vi "SCE_create_border.vi"(7 "VIC-II":T1, 11 "screen in":picture) -> (3 "screen out":picture)   [LabVIEW 2018]
uses:
  SCE_VIC-II_registry.ctl
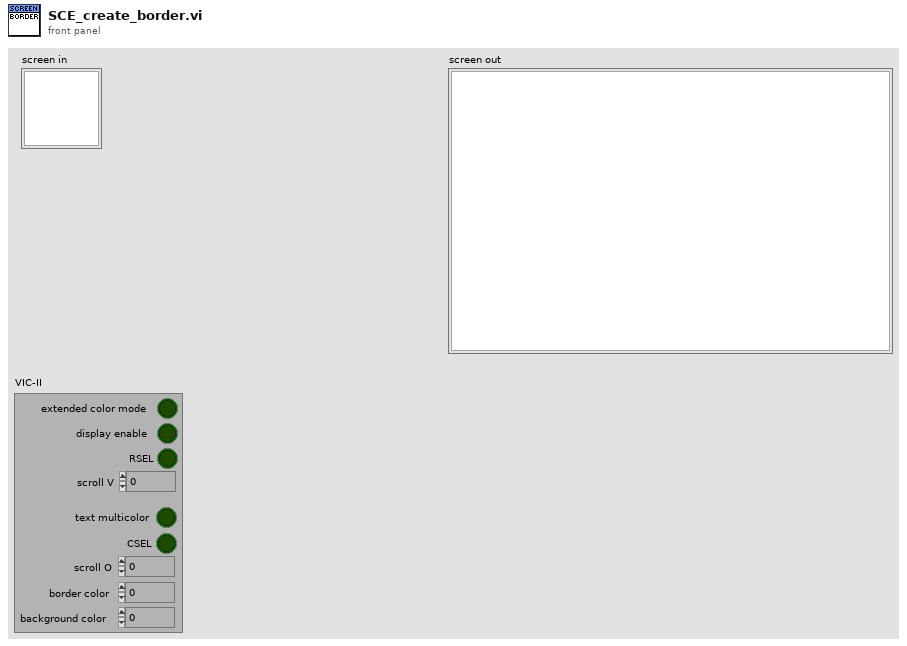
[diagram p1: front panel]
types:
  T1 = typedef "SCE_VIC-II_registry.ctl" = cluster{"extended color mode":bool, "display enable":bool, "RSEL":bool, "scroll V":u8, "text multicolor":bool, "CSEL":bool, "scroll O":u8, "border color":u8, "background color":u8}
  T2 = cluster{"left":i16, "top":i16, "right":i16, "bottom":i16}
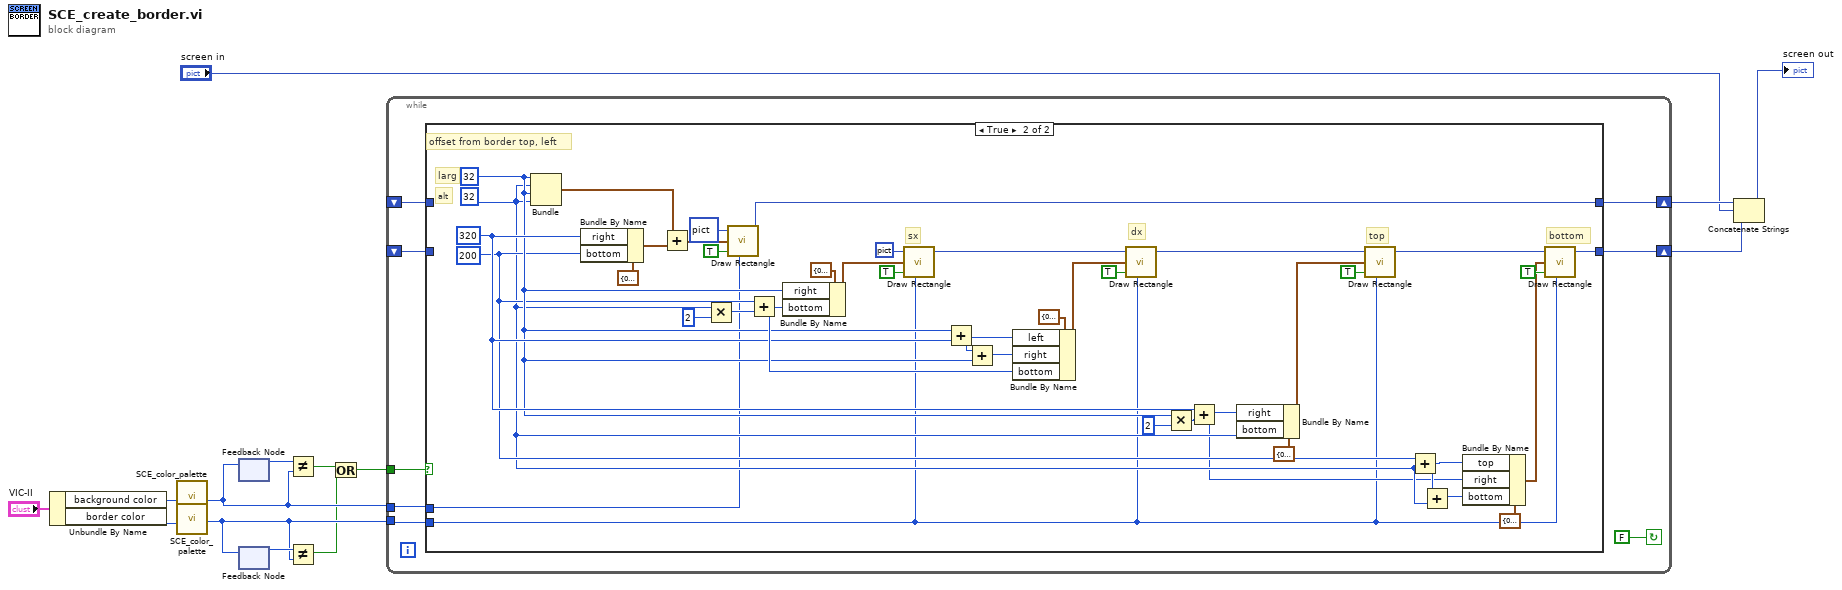
[diagram p0: block diagram]
diagram:
  n1 = Unbundle By Name("VIC-II") -> ("background color"=w13:u8, "border color"=w12:u8)
  n2 = call "SCE_color_palette.vi"("color index"=w13) -> ("selected color"=w6:u32)  [unwired: 9 in, 1 out]
  n3 = call "SCE_color_palette.vi"("color index"=w12) -> ("selected color"=w4:u32)  [unwired: 9 in, 1 out]
  n4 = feedback-in #1(w6) -> ()
  n5 = feedback #1() -> (w7:u32)  [unwired: 1 in]
  n6 = feedback #2() -> (w5:u32)  [unwired: 1 in]
  n7 = feedback-in #2(w4) -> ()
  n8 = Not Equal?(x=w7, y=w6) -> (x != y?=w3:bool)
  n9 = Not Equal?(x=w5, y=w4) -> (x != y?=w2:bool)
  n10 = Or(x=w3, y=w2) -> (x .or. y?=w1:bool)
  n11 = while {
    tunnel: w6 -> [w20]
    tunnel: w4 -> [w19]
    shift-right: [w22] -> w11
    shift-left: _ -> [w16]
    shift-right: [w21] -> w8
    shift-left: _ -> [w15]
    tunnel: w1 -> [w17]
    stop <- FALSE continue-if-true
    n12 = case shown="True" w17 {
      tunnel: [w24 w61] -> w22
      tunnel: [w23 w27] -> w21
      tunnel: w20 -> [_ w26]
      tunnel: w19 -> [_ w25]
      tunnel: w16 -> [w24 _]
      tunnel: w15 -> [w23 _]
      frame False {
      }
      frame True {
        w43 = i16 320 ("right")
        w32 = i16 200 ("bottom")
        w30 = i16 32 ("x")
        w40 = i16 32 ("x")
        # "bottom"
        # "top"
        # "dx"
        # "sx"
        # "alt"
        # "larg"
        # "offset from border top, left"
        n13 = Bundle("x"=w40, "x"=w30, "x"=w40, "x"=w30) -> (w64:cluster{"x":i16, "x":i16, "x":i16, "x":i16})  [unwired: 1 in]
        n14 = Bundle By Name(cluster=T2 {"left"=0, "top"=0, "right"=320, "bottom"=200} ("rect"), "right"=w43, "bottom"=w32) -> (w58:T2)
        n15 = Add(x=w64, y=w58) -> (x+y=w63:cluster{i16, i16, i16, i16})
        n16 = Multiply(x=w30, y=i16 2) -> (x*y=w47:i16)
        n17 = call <vilib>:"Draw Rectangle.vi"("picture"=picture data[5B], "rect"=w63, "fill?(F)"=TRUE, "color(black)"=w26) -> ("new picture"=w61:picture)  [unwired: 5 in]
        n18 = Add(x=w32, y=w47) -> (x+y=w45:i16)
        n19 = Bundle By Name(cluster=T2 {"left"=0, "top"=0, "right"=320, "bottom"=200} ("rect"), "right"=w40, "bottom"=w45) -> (w56:T2)
        n20 = call <vilib>:"Draw Rectangle.vi"("picture"=picture data[5B], "rect"=w56, "fill?(F)"=TRUE, "color(black)"=w25) -> ("new picture"=w50:picture)  [unwired: 5 in]
        n21 = Add(x=w40, y=w43) -> (x+y=w49:i16)
        n22 = Add(x=w49, y=w40) -> (x+y=w48:i16)
        n23 = Bundle By Name(cluster=T2 {"left"=0, "top"=0, "right"=320, "bottom"=200} ("rect"), "left"=w49, "right"=w48, "bottom"=w45) -> (w52:T2)
        n24 = call <vilib>:"Draw Rectangle.vi"("picture"=w50, "rect"=w52, "fill?(F)"=TRUE, "color(black)"=w25) -> ("new picture"=w37:picture)  [unwired: 5 in]
        n25 = Multiply(x=w40, y=i16 2) -> (x*y=w41:i16)
        n26 = Add(x=w43, y=w41) -> (x+y=w28:i16)
        n27 = Bundle By Name(cluster=T2 {"left"=0, "top"=0, "right"=320, "bottom"=200} ("rect"), "right"=w28, "bottom"=w30) -> (w39:T2)
        n28 = call <vilib>:"Draw Rectangle.vi"("picture"=w37, "rect"=w39, "fill?(F)"=TRUE, "color(black)"=w25) -> ("new picture"=w35:picture)  [unwired: 5 in]
        n29 = Add(x=w32, y=w30) -> (x+y=w31:i16)
        n30 = Add(x=w31, y=w30) -> (x+y=w29:i16)
        n31 = Bundle By Name(cluster=T2 {"left"=0, "top"=0, "right"=320, "bottom"=200} ("rect"), "top"=w31, "right"=w28, "bottom"=w29) -> (w33:T2)
        n32 = call <vilib>:"Draw Rectangle.vi"("picture"=w35, "rect"=w33, "fill?(F)"=TRUE, "color(black)"=w25) -> ("new picture"=w27:picture)  [unwired: 5 in]
      }
    }
  }
  n33 = Concatenate Strings(w11, "screen in", w8) -> (→"screen out":picture)
